vi "odczyt_logow_z_MCU.vi"(11 "read buffer in":string) -> (2 "read buffer out":string, 3 "Boolean":bool)   [LabVIEW 2025]
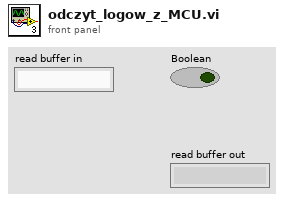
[diagram p1: front panel]
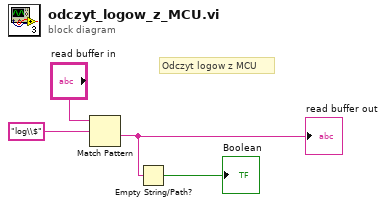
[diagram p0: block diagram]
diagram:
  # "Odczyt logow z MCU"
  n1 = Match Pattern(string="read buffer in", regular expression="log\\$") -> (after substring=w3:string)  [unwired: 1 in, 3 out]
  "read buffer out" <- w3
  n2 = Empty String/Path?(string/path=w3) -> (empty?=→"Boolean":bool)
